vi "ICA_16_Potluri.vi"() -> ()   [LabVIEW 2016]
uses:
  <vilib>/NXT/Block Support/NXT_OutputPort.ctl
  <vilib>/NXT/Dual Mode Library/Sensors/EV3_Ultrasonic_CM.vi
  <vilib>/NXT/NXTIO Xnodes/NXTIONodeSubVIs/LEGOMoveAllMotors.vi
  <vilib>/NXT/Dual Mode Library/Waits/Wait_Num.vi
  <vilib>/NXT/NXTIO Xnodes/NXTIONodeSubVIs/LEGOMoveAllMotorsDistance.vi
  <vilib>/NXT/NXTIO Xnodes/NXTIONodeSubVIs/NXTMotorRunDistance.vi
  <vilib>/NXT/NXTIO Xnodes/NXTIONodeSubVIs/LEGOStopAllMotors.vi
  <vilib>/NXT/Subs/LVHSConnector.ctl
  <vilib>/NXT/NXTIO Xnodes/NXTIOXNode/NXTIO.xnode
  <vilib>/NXT/NXTIO Xnodes/AddressXNode/NXTIOAddress.xnode
  <vilib>/NXT/LegoClasses/BrickReference/BrickReference.lvclass
panel:
  out "Numeric":dbl
  out "Numeric 2":dbl
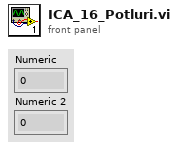
[diagram p1: front panel]
types:
  T1 = typedef "LVHSConnector.ctl" = refnum<class "BrickReference.lvclass">
  T2 = typedef "NXT_OutputPort.ctl" = u8
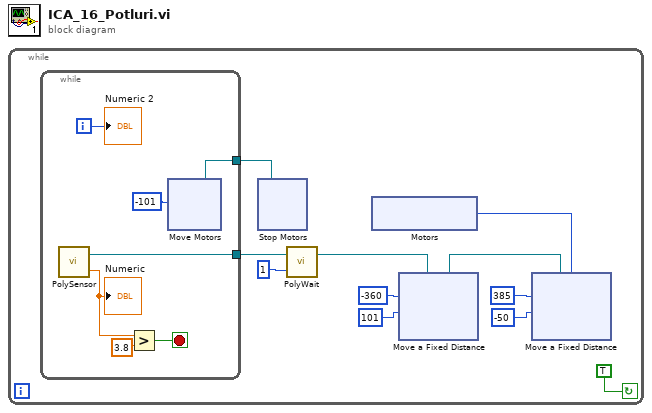
[diagram p0: block diagram]
diagram:
  n1 = while {
    stop <- TRUE continue-if-true
    n2 = while {
      tunnel: [w39] -> w5
      tunnel: [w38] -> w2
      i -> [w40]
      stop <- w43 stop-if-true
      n3 = call-poly <vilib>:"PolySensor.vi"() -> ("Centimeters"=w41:sgl, "NXT/EV3"=w39:T1)  [unwired: 3 in]
      "Numeric" <- w41
      n4 = Greater?(x=w41, y=3.8) -> (0:w43:bool)
      n5 = xnode "Move Motors"("Power/Speed 1"=-101) -> ("NXT/EV3"=w38:T1)  [unwired: 2 in]
      "Numeric 2" <- w40
    }
    n6 = xnode "Stop Motors"("NXT/EV3"=w2) -> ()  [unwired: 1 in, 1 out]
    n7 = call-poly <vilib>:"PolyWait.vi"("Time (1 sec)"=1, "NXT/EV3"=w5) -> ("NXT/EV3"=w4:T1)  [unwired: 2 in]
    n8 = xnode "Motors"() -> ("Motor"=w7:T2)
    n9 = xnode "Move a Fixed Distance"("Speed 1"=101, "Distance 1"=-360, "NXT/EV3"=w4) -> ("NXT/EV3"=w6:T1)  [unwired: 1 in]
    n10 = xnode "Move a Fixed Distance"("Speed 1"=-50, "Distance 1"=385, "Motors"=w7, "NXT/EV3"=w6) -> ()  [unwired: 1 out]
  }
